vi "TCPWrite.vi"(8 "error in":errorcluster, 10 "data in":string, 11 "StructIn":T1) -> (0 "error out":errorcluster, 1 "WroteAll?":bool, 3 "StructOut":T1)   [LabVIEW 2021, in "LibDan.lvlib"]
uses:
  LibDan.lvlib
  TerminalDef.ctl
  <vilib>/Utility/config.llb/Config Data RefNum.ctl
  <vilib>/Utility/config.llb/NI_LVConfig.lvlib
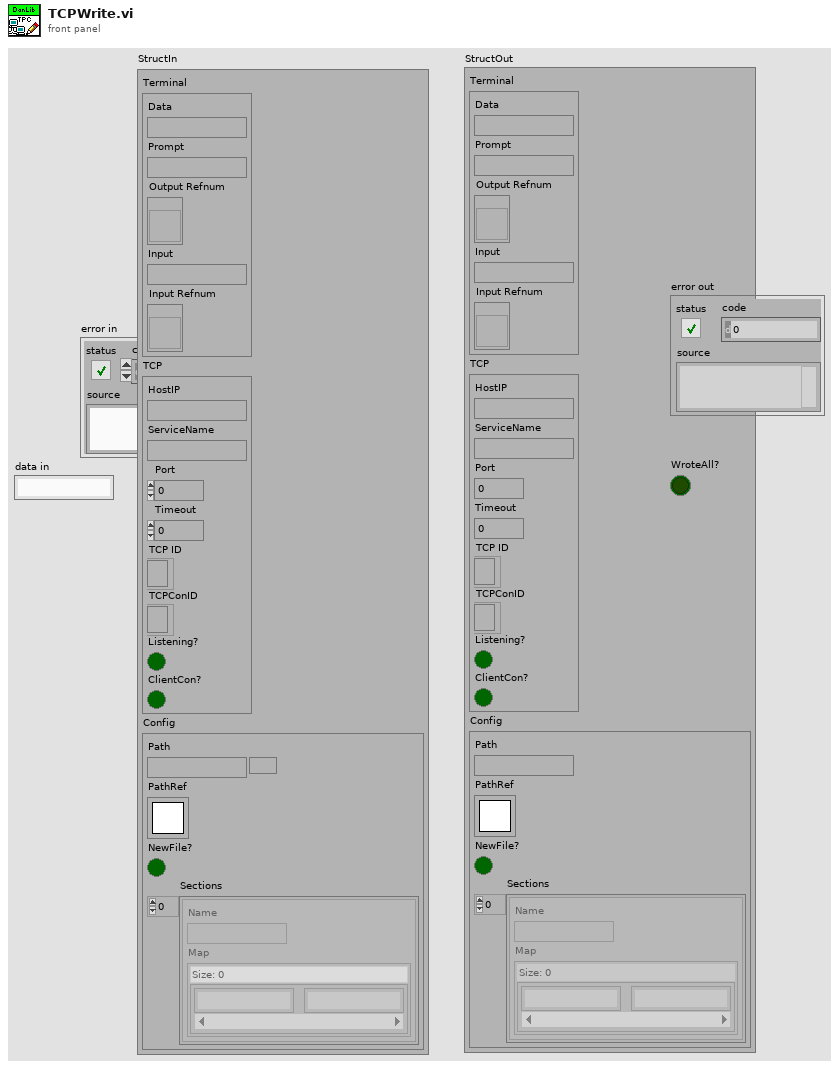
[diagram p1: front panel]
types:
  T1 = typedef "LibDan.lvlib/TerminalDef.ctl" = cluster{"Terminal":cluster{"Data":string, "Prompt":string, "Output Refnum":refnum<vi>, "Input":string, "Input Refnum":refnum<vi>}, "TCP":cluster{"HostIP":string, "ServiceName":string, "Port":u16, "Timeout":i32, "TCP ID":refnum<k5>, "TCPConID":refnum<k5>, "Listening?":bool, "ClientCon?":bool}, "Config":cluster{"Path":path, "PathRef":T2, "NewFile?":bool, "Sections":cluster{"Name":string, "Map":map{string, string}}[]}}
  T2 = typedef "NI_LVConfig.lvlib/Config Data RefNum.ctl" = refnum<k1>
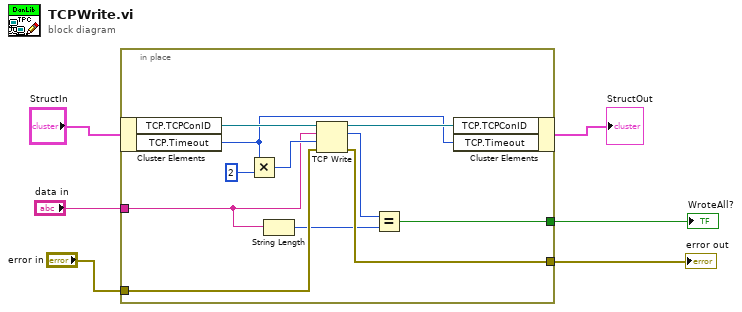
[diagram p0: block diagram]
diagram:
  n1 = in-place {
    in-place-border: "error in" -> [w17]
    in-place-border: [w15] -> w3
    in-place-border: "data in" -> [w10]
    in-place-border: [w7] -> w1
    n2 = in-place-cluster #1("StructIn") -> ("TCP.TCPConID"=w14:refnum<k5>, "TCP.Timeout"=w11:i32)
    n3 = Multiply(x=w11, y=2) -> (x*y=w12:i32)
    n4 = String Length(string=w10) -> (length=w8:i32)
    n5 = TCP Write(connection ID=w14, data in=w10, error in (no error)=w17, 9:w12) -> (connection ID out=w16:refnum<k5>, bytes written=w9:i32, error out=w15:errorcluster)
    n6 = Equal?(x=w9, y=w8) -> (x = y?=w7:bool)
    n7 = in-place-cluster #1("TCP.TCPConID"=w16, "TCP.Timeout"=w11) -> (→"StructOut":T1)
  }
  "error out" <- w3
  "WroteAll?" <- w1
